vi "generateDataRequestMessage.vi"(8 "error in (no error)":errorcluster, 11 "ILCSim1 in":refnum<class "ILCSim1.lvclass">) -> (0 "error out":errorcluster, 3 "ILCSim1 out":refnum<class "ILCSim1.lvclass">)   [LabVIEW 2013, in "ILCSim1.lvclass"]
uses:
  ILCSim1.lvclass
  ILCSimulatorSignals/RequestParameters.ctl
  <userlib>/Common/ILC/Configuration/ScanRate_Hz_MultichannelOptions.ctl
  ILCSim1.lvclass/ILCSim1.ctl
  <userlib>/Common/ILC/Configuration/ILCConfiguration.lvlib
  ILCSimulatorSignals/ILCSimulatorSignals.lvlib
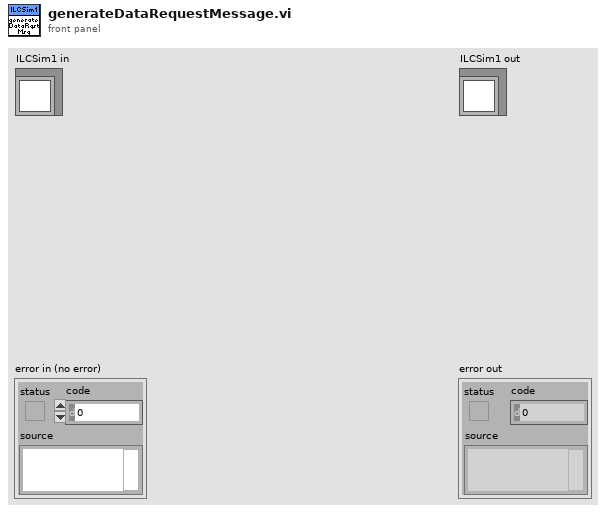
[diagram p1: front panel]
types:
  T1 = typedef "ILCSimulatorSignals.lvlib/RequestParameters.ctl" = cluster{"Time Stamp":timestamp, "answeredIsTrue":bool, "Scan Rate (Hz) ":T2, "Input Channels":enum16{"Channel 0", "3 Channels", "5 Channels"}}
  T2 = typedef "ILCCommon.lvlib/ILCConfiguration.lvlib/ScanRate_Hz_MultichannelOptions.ctl" = enum16{"50", "60", "100", "120", "200", "240", "300", "400", "480", "600", "1200", "2400", "4800"}
  T3 = typedef "ILCCommon.lvlib/ILCConfiguration.lvlib/InputChannels.ctl" = enum16{"Channel 0", "3 Channels", "5 Channels"}
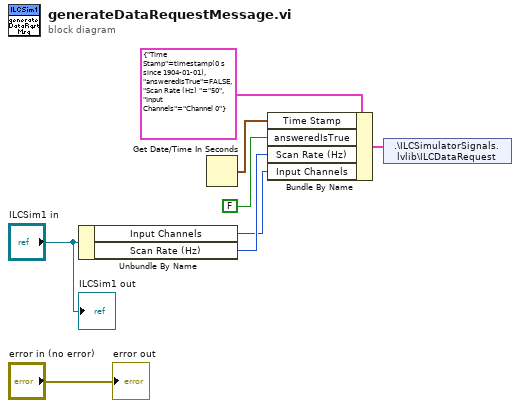
[diagram p0: block diagram]
diagram:
  n1 = Unbundle By Name("ILCSim1 in") -> ("Input Channels"=w7:T3, "Scan Rate (Hz)"=w8:T2)
  n2 = Get Date/Time In Seconds() -> (seconds since 1Jan1904=w4:timestamp)
  n3 = Bundle By Name(cluster=T1 {"Time Stamp"=timestamp(0 s since 1904-01-01), "answeredIsTrue"=FALSE, "Scan Rate (Hz) "=enum."50", "Input Channels"=enum."Channel 0"} ("ILCDataRequest"), "Time Stamp"=w4, "answeredIsTrue"=FALSE, "Scan Rate (Hz)"=w8, "Input Channels"=w7) -> (w5:T1)
  n4 = shared-variable ".\\ILCSimulatorSignals.lvlib\\ILCDataRequest"(w5) -> ()  [unwired: 1 in, 1 out]
  "error out" <- "error in (no error)"
  "ILCSim1 out" <- "ILCSim1 in"
